vi "Update Indicators.vi"(8 "error in (no error)":errorcluster) -> (0 "error out":errorcluster)   [LabVIEW 2018]
uses:
  CTL/FGV - R-W.ctl
panel:
  out "Cmd Out":bool[](array[boolean])
  out "Lamp FB":bool[](array[boolean])
  out "Flash FB":bool[](array[boolean])
  in  "Lamp Reference":refnum<vi>
  out "Fault FB":bool[](array[boolean])
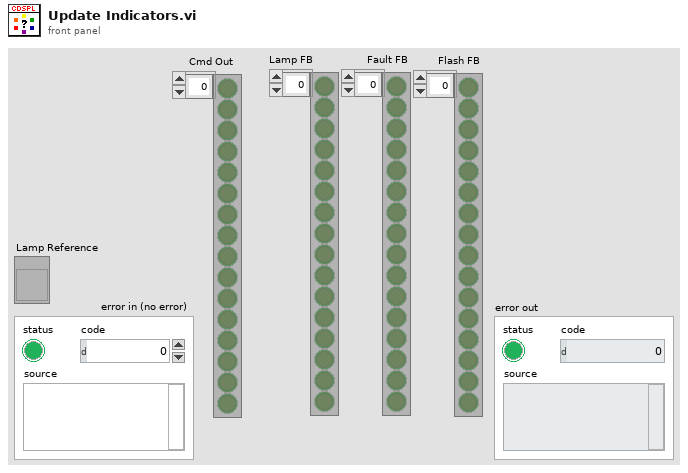
[diagram p1: front panel]
types:
  T1 = typedef "FGV - R-W.ctl" = enum16{"W", "R"}
  T2 = typedef "Lamp Ref.ctl" = refnum<vi>[]
  T3 = enum16{"ON State", "OFF State", "FAULTY", "Fault Flash", "Nothing"}
  T4 = enum8{"Enabled", "Disabled", "Disabled and Grayed Out"}
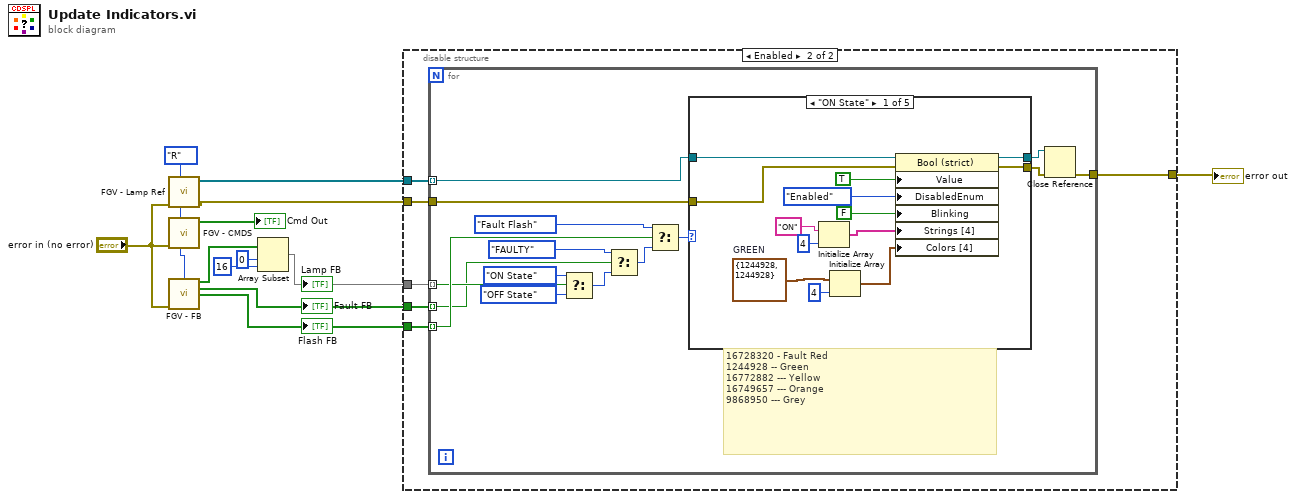
[diagram p0: block diagram]
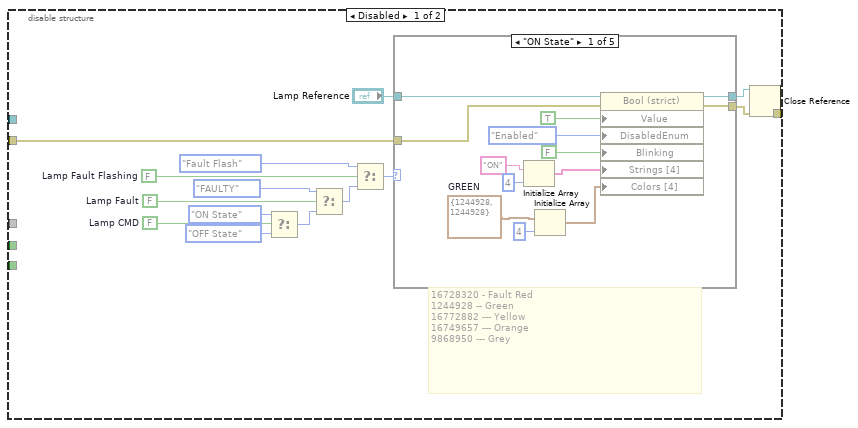
[diagram p2: hidden frame]
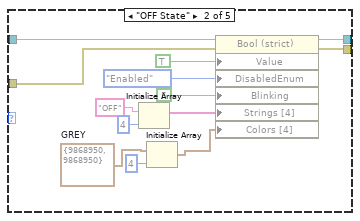
[diagram p3: hidden frame]
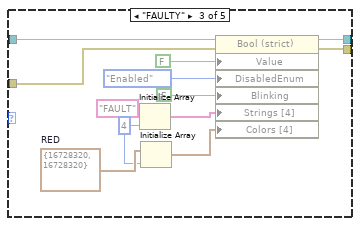
[diagram p4: hidden frame]
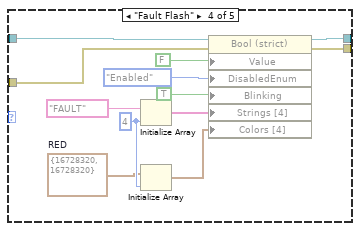
[diagram p5: hidden frame]
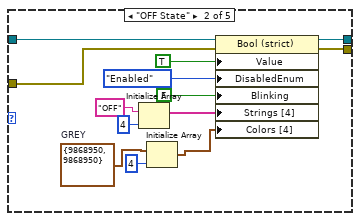
[diagram p7: hidden frame]
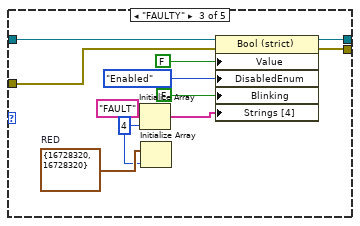
[diagram p8: hidden frame]
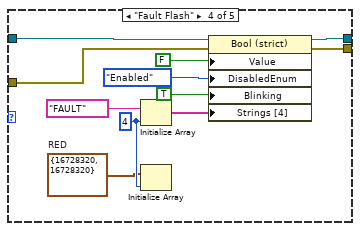
[diagram p9: hidden frame]
diagram:
  w9 = FGV_-_R-W."R" ("Action")
  n1 = call "FGV - Lamp Ref.vi"("Action"=w9, "error in (no error)"="error in (no error)") -> ("error out"=w7:errorcluster, "Lamp Ref Out"=w6:T2)  [unwired: 8 in]
  n2 = call "FGV - CMDS.vi"("Action"=w9, "error in (no error)"="error in (no error)") -> ("Cmd Out"=→"Cmd Out":bool[])  [unwired: 8 in, 1 out]
  n3 = call "FGV - FB.vi"("Action"=w9, "error in (no error)"="error in (no error)") -> ("CMD FB"=w1:bool[], "Fault FB"=w3:bool[], "Flash FB"=w5:bool[])  [unwired: 7 in, 4 out]
  "Fault FB" <- w3
  "Flash FB" <- w5
  n4 = Array Subset(array=w1, index=0, length=16) -> (w4:bool[])
  "Lamp FB" <- w4
  n5 = disable-structure shown="Enabled" {
    disable-tunnel: w7 -> [w14 w85]
    disable-tunnel: w6 -> [_ w84]
    disable-tunnel: w5 -> [_ w83]
    disable-tunnel: w4 -> [_ w82]
    disable-tunnel: w3 -> [_ w81]
    disable-tunnel: [w13 w80] -> w2
    frame Disabled {
      w19 = FALSE  # Lamp Fault
      w16 = FALSE  # Lamp CMD
      w24 = FALSE  # Lamp Fault Flashing
      # "16728320 - Fault Red\n1244928 -- Green\n16772882 --- Yellow\n16749657 --- Orange\n9868950 --- Grey"
      n6 = Select(t=T3."ON State", s=w16, f=T3."OFF State" ("State")) -> (s? t:f=w20:T3)
      n7 = Select(t=T3."FAULTY", s=w19, f=w20) -> (s? t:f=w23:T3)
      n8 = Select(t=T3."Fault Flash", s=w24, f=w23) -> (s? t:f=w15:T3)
      n9 = case shown="\"ON State\"" w15 {
        tunnel: "Lamp Reference" -> [w40 w53 w65 w77 w79]
        tunnel: w14 -> [w39 w52 w64 w76 w78]
        tunnel: [w35 w48 w60 w72 w79] -> w27
        tunnel: [w34 w47 w59 w71 w78] -> w26
        frame "ON State" {
          w29 = cluster{"Numeric":i32, "Numeric":i32} {"Numeric"=1244928, "Numeric"=1244928}  # GREEN
          n10 = Initialize Array("ON" ("String"), 4 ("dimension size")) -> (w31:string[])
          n11 = Initialize Array(w29, 4 ("dimension size")) -> (w28:cluster{"Numeric":i32, "Numeric":i32}[])
          n12 = property class="Bool (strict)"(reference=w40, error in=w39, "Value"=TRUE, "DisabledEnum"=T4."Enabled" ("Disabled"), "Blinking"=FALSE, "Strings [4]"=w31, "Colors [4]"=w28) -> (reference out=w35:refnum<vi>, error out=w34:errorcluster)
        }
        frame "OFF State" {
          w42 = cluster{"Numeric":i32, "Numeric":i32} {"Numeric"=9868950, "Numeric"=9868950}  # GREY
          n13 = Initialize Array("OFF" ("String"), 4 ("dimension size")) -> (w44:string[])
          n14 = Initialize Array(w42, 4 ("dimension size")) -> (w41:cluster{"Numeric":i32, "Numeric":i32}[])
          n15 = property class="Bool (strict)"(reference=w53, error in=w52, "Value"=TRUE, "DisabledEnum"=T4."Enabled" ("Disabled"), "Blinking"=FALSE, "Strings [4]"=w44, "Colors [4]"=w41) -> (reference out=w48:refnum<vi>, error out=w47:errorcluster)
        }
        frame "FAULTY" {
          w56 = cluster{"Numeric":i32, "Numeric":i32} {"Numeric"=16728320, "Numeric"=16728320}  # RED
          w55 = 4 ("dimension size")
          n16 = Initialize Array("FAULT" ("String"), w55) -> (w57:string[])
          n17 = Initialize Array(w56, w55) -> (w54:cluster{"Numeric":i32, "Numeric":i32}[])
          n18 = property class="Bool (strict)"(reference=w65, error in=w64, "Value"=FALSE, "DisabledEnum"=T4."Enabled" ("Disabled"), "Blinking"=FALSE, "Strings [4]"=w57, "Colors [4]"=w54) -> (reference out=w60:refnum<vi>, error out=w59:errorcluster)
        }
        frame "Fault Flash" {
          w67 = cluster{"Numeric":i32, "Numeric":i32} {"Numeric"=16728320, "Numeric"=16728320}  # RED
          w68 = 4 ("dimension size")
          n19 = Initialize Array("FAULT" ("String"), w68) -> (w69:string[])
          n20 = Initialize Array(w67, w68) -> (w66:cluster{"Numeric":i32, "Numeric":i32}[])
          n21 = property class="Bool (strict)"(reference=w77, error in=w76, "Value"=FALSE, "DisabledEnum"=T4."Enabled" ("Disabled"), "Blinking"=TRUE, "Strings [4]"=w69, "Colors [4]"=w66) -> (reference out=w72:refnum<vi>, error out=w71:errorcluster)
        }
        frame "Nothing" {
        }
      }
      n22 = Close Reference(reference=w27, error in (no error)=w26) -> (error out=w13:errorcluster)
    }
    frame Enabled {
      n23 = for {
        tunnel: w85 -> [w91]
        tunnel: w84 -> [w90] mode=indexing
        tunnel: w83 -> [w89] mode=indexing
        tunnel: w82 -> [w88] mode=indexing
        tunnel: w81 -> [w87] mode=indexing
        tunnel: [w86] -> w80
        # "16728320 - Fault Red\n1244928 -- Green\n16772882 --- Yellow\n16749657 --- Orange\n9868950 --- Grey"
        n24 = Select(t=T3."ON State", s=w88, f=T3."OFF State" ("State")) -> (s? t:f=w95:T3)
        n25 = Select(t=T3."FAULTY", s=w87, f=w95) -> (s? t:f=w98:T3)
        n26 = Select(t=T3."Fault Flash", s=w89, f=w98) -> (s? t:f=w92:T3)
        n27 = case shown="\"ON State\"" w92 {
          tunnel: w90 -> [w113 w126 w137 w148 w150]
          tunnel: w91 -> [w112 w125 w136 w147 w149]
          tunnel: [w108 w121 w132 w143 w150] -> w100
          tunnel: [w107 w120 w131 w142 w149] -> w99
          frame "ON State" {
            w102 = cluster{"Numeric":i32, "Numeric":i32} {"Numeric"=1244928, "Numeric"=1244928}  # GREEN
            n28 = Initialize Array("ON" ("String"), 4 ("dimension size")) -> (w104:string[])
            n29 = Initialize Array(w102, 4 ("dimension size")) -> (w101:cluster{"Numeric":i32, "Numeric":i32}[])
            n30 = property class="Bool (strict)"(reference=w113, error in=w112, "Value"=TRUE, "DisabledEnum"=T4."Enabled" ("Disabled"), "Blinking"=FALSE, "Strings [4]"=w104, "Colors [4]"=w101) -> (reference out=w108:refnum<vi>, error out=w107:errorcluster)
          }
          frame "OFF State" {
            w115 = cluster{"Numeric":i32, "Numeric":i32} {"Numeric"=9868950, "Numeric"=9868950}  # GREY
            n31 = Initialize Array("OFF" ("String"), 4 ("dimension size")) -> (w117:string[])
            n32 = Initialize Array(w115, 4 ("dimension size")) -> (w114:cluster{"Numeric":i32, "Numeric":i32}[])
            n33 = property class="Bool (strict)"(reference=w126, error in=w125, "Value"=TRUE, "DisabledEnum"=T4."Enabled" ("Disabled"), "Blinking"=FALSE, "Strings [4]"=w117, "Colors [4]"=w114) -> (reference out=w121:refnum<vi>, error out=w120:errorcluster)
          }
          frame "FAULTY" {
            w128 = cluster{"Numeric":i32, "Numeric":i32} {"Numeric"=16728320, "Numeric"=16728320}  # RED
            w127 = 4 ("dimension size")
            n34 = Initialize Array("FAULT" ("String"), w127) -> (w129:string[])
            n35 = Initialize Array(w128, w127) -> ()  [unwired: 1 out]
            n36 = property class="Bool (strict)"(reference=w137, error in=w136, "Value"=FALSE, "DisabledEnum"=T4."Enabled" ("Disabled"), "Blinking"=FALSE, "Strings [4]"=w129) -> (reference out=w132:refnum<vi>, error out=w131:errorcluster)
          }
          frame "Fault Flash" {
            w138 = cluster{"Numeric":i32, "Numeric":i32} {"Numeric"=16728320, "Numeric"=16728320}  # RED
            w139 = 4 ("dimension size")
            n37 = Initialize Array("FAULT" ("String"), w139) -> (w140:string[])
            n38 = Initialize Array(w138, w139) -> ()  [unwired: 1 out]
            n39 = property class="Bool (strict)"(reference=w148, error in=w147, "Value"=FALSE, "DisabledEnum"=T4."Enabled" ("Disabled"), "Blinking"=TRUE, "Strings [4]"=w140) -> (reference out=w143:refnum<vi>, error out=w142:errorcluster)
          }
          frame "Nothing" {
          }
        }
        n40 = Close Reference(reference=w100, error in (no error)=w99) -> (error out=w86:errorcluster)
      }
    }
  }
  "error out" <- w2
